vi "Set message.vi"(10 "WampMessage MsgPack":refnum<class "WampMessage MsgPack.lvclass">, 11 "EventHandler MsgPack in":refnum<class "EventHandler MsgPack.lvclass">) -> (3 "EventHandler MsgPack out":refnum<class "EventHandler MsgPack.lvclass">)   [LabVIEW 2020, in "wamplv.lvlib" / "EventHandler MsgPack.lvclass"]
uses:
  EventHandler MsgPack.lvclass
  EventHandler MsgPack.lvclass/EventHandler MsgPack.ctl
  SerialisedMessages/MsgPackMessage/WampMessage MsgPack.lvclass
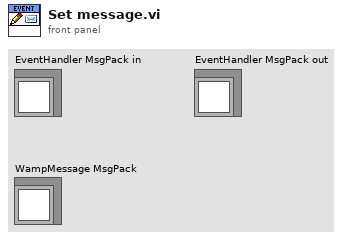
[diagram p1: front panel]
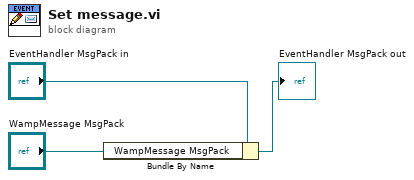
[diagram p0: block diagram]
diagram:
  n1 = Bundle By Name(cluster="EventHandler MsgPack in", "WampMessage MsgPack"="WampMessage MsgPack") -> (→"EventHandler MsgPack out":refnum<class "EventHandler MsgPack.lvclass">)
